vi "Set input current_ChQ.vi"(0 "channel name":string, 3 "4070_address":refnum<k15>="PXI3Slot5_5 (8)" caption="4070_out", 4 "res(input)":dbl=110.0, 6 "the optimum current(input)":dbl format="%#_6f", 7 "accuracy (input)":dbl step=0.01, 8 "instrument handle":refnum<k15>, 9 "the upper limit for the voltage":dbl=5.0, 10 "Start voltage":dbl=3.0 format="%#.7f", 11 "the lower limit for the voltage":dbl=1.0) -> (1 "current value, mA":dbl, 2 "Error message":string, 5 "accommodated voltage (out)":dbl)   [LabVIEW 2013]
uses:
  <instrlib>/niDMM/nidmm.llb/niDMM Resolution in Digits.ctl
  <instrlib>/niDMM/nidmm.llb/niDMM Function.ctl
  <vilib>/Analysis/baseanly.llb/Mean (DBL).vi
  <instrlib>/niDMM/nidmm.llb/niDMM Configure Measurement Digits.vi
  <vilib>/Analysis/NI_AALBase.lvlib
panel:
  out "CH1_Uпит, mA":dbl=15.418111291908591 caption="CH1_AO, ìA" format="%_6g"
  out "the voltage drop across the resistor":dbl=1.1
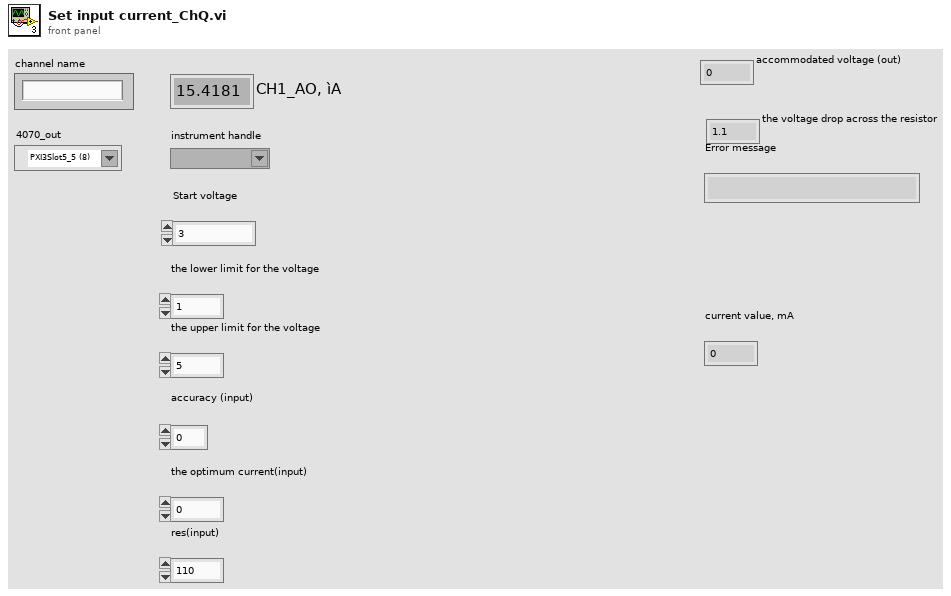
[diagram p1: front panel]
types:
  T1 = typedef "niDMM Function.ctl" = enum16{"DC Volts", "AC Volts", "DC Current", "AC Current", "2-wire Resistance", "4-wire Resistance", "Diode", "Frequency", "Period", "AC Volts DC Coupled", "Capacitance", "Inductance", "Temperature"}
  T2 = typedef "niDMM Resolution in Digits.ctl" = dbl
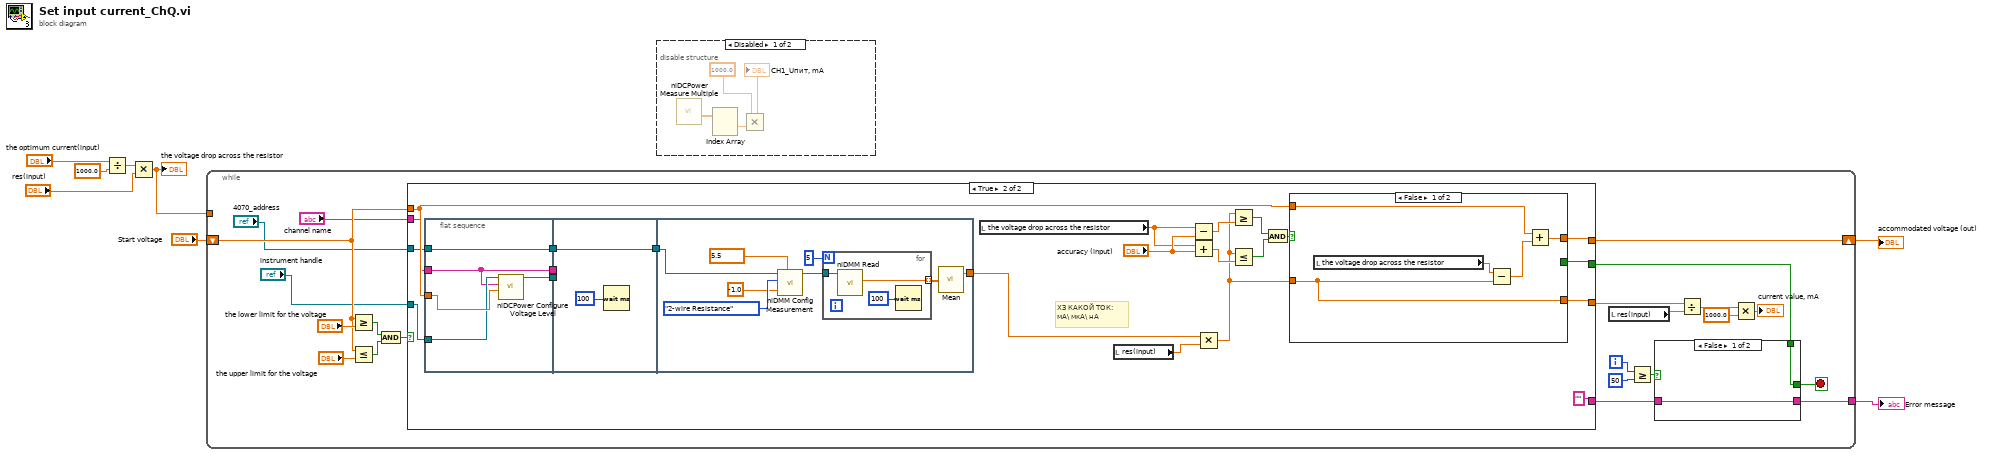
[diagram p0: block diagram]
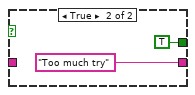
[diagram p3: hidden frame]
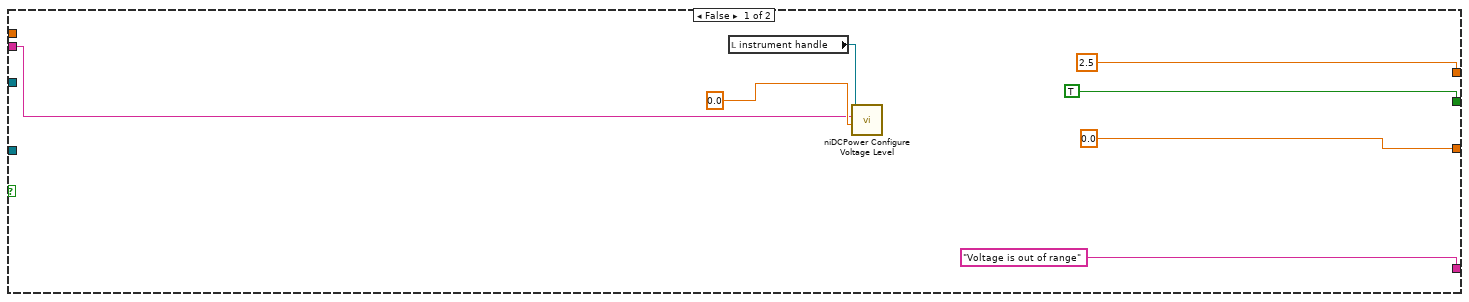
[diagram p4: hidden frame]
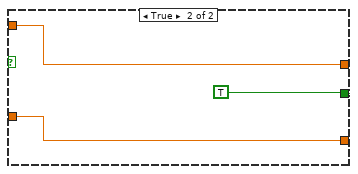
[diagram p5: hidden frame]
diagram:
  n1 = Divide(x="the optimum current(input)", y=1000.0) -> (x/y=w5:dbl)
  n2 = Multiply(x=w5, y="res(input)") -> (x*y=w1:dbl)
  "the voltage drop across the resistor" <- w1
  n3 = while {
    tunnel: [w14] -> w8
    shift-right: [w20] -> w2
    shift-left: "Start voltage" -> [w21]
    tunnel: w1 -> [_]
    i -> [w17]
    stop <- w13 stop-if-true
    n4 = Greater Or Equal?(x=w21, y="the lower limit for the voltage") -> (x >= y?=w29:bool)
    n5 = Less Or Equal?(x=w21, y="the upper limit for the voltage") -> (x <= y?=w30:bool)
    n6 = And(x=w29, y=w30) -> (x .and. y?=w26:bool)
    n7 = case shown="True" w26 {
      tunnel: ["Voltage is out of range" ""] -> w15
      tunnel: [2.5 ("accommodated voltage") w55] -> w20
      tunnel: [TRUE w61] -> w12
      tunnel: [0.0 w56] -> w19
      tunnel: w21 -> [_ w51]
      tunnel: "instrument handle" -> [_ w47]
      tunnel: "channel name" -> [w35 w46]
      tunnel: "4070_address" -> [_ w44]
      frame False {
        n8 = local read "instrument handle"() -> (w37:refnum<k15>)
        n9 = call <instrlib>:"niDCPower Configure Voltage Level.vi"("voltage level"=0.0, "channel name"=w35, "instrument handle"=w37) -> ()  [unwired: 7 in, 2 out]
      }
      frame True {
        # "ХЗ КАКОЙ ТОК:\nмА\\ мкА\\ нА"
        n10 = flat-sequence {
          tunnel: w51 -> [w67]
          tunnel: [w68] -> w52
          tunnel: [w65] -> w48
          tunnel: w47 -> [w66]
          tunnel: w46 -> [w65]
          tunnel: [w64] -> w45
          tunnel: w44 -> [w64]
          tunnel: w52 -> [_]
          tunnel: w48 -> [_]
          tunnel: w45 -> [w69]
          tunnel: [w69] -> w43
          tunnel: w43 -> [w72]
          tunnel: [w71] -> w42
          frame #0 {
            n11 = call <instrlib>:"niDCPower Configure Voltage Level.vi"("voltage level"=w67, "channel name"=w65, "instrument handle"=w66) -> ("instrument handle out"=w68:refnum<k15>)  [unwired: 7 in, 1 out]
          }
          frame #1 {
            n12 = Wait (ms)(milliseconds to wait=u32 100) -> ()  [unwired: 1 out]
          }
          frame #2 {
            w75 = T2 5.5 items=["3 1/2"=3.5, "4 1/2"=4.5, "5 1/2"=5.5, "6 1/2"=6.5, "7 1/2"=7.5] ("Resolution in Digits")
            n13 = call-poly <instrlib>:"niDMM Config Measurement.vi"("Range"=-1.0 ("Configuration:Measurement Options:Max Frequency"), "Resolution in Digits"=w75, "Function"=niDMM_Function."2-wire Resistance" ("multimeter mode"), "instrument handle"=w72) -> ("instrument handle out"=w76:refnum<k15>)  [unwired: 6 in, 1 out]
            n14 = for {
              N: 5 -> [_]
              tunnel: w76 -> [w80]
              tunnel: [w79] -> w77 mode=indexing
              n15 = call <instrlib>:"niDMM Read.vi"("instrument handle"=w80) -> ("Measurement"=w79:dbl)  [unwired: 8 in, 2 out]
              n16 = Wait (ms)(milliseconds to wait=u32 100) -> ()  [unwired: 1 out]
            }
            n17 = call-poly <vilib>:"Mean.vi"("X"=w77) -> ("mean"=w71:dbl)  [unwired: 1 out]
          }
        }
        n18 = local read "the voltage drop across the resistor"() -> (w59:dbl)
        n19 = local read "res(input)"() -> (w50:dbl)
        n20 = Subtract(x=w59, y="accuracy (input)") -> (x-y=w63:dbl)
        n21 = Add(x=w59, y="accuracy (input)") -> (x+y=w62:dbl)
        n22 = Multiply(x=w42, y=w50) -> (x*y=w49:dbl)
        n23 = Greater Or Equal?(x=w49, y=w63) -> (x >= y?=w57:bool)
        n24 = Less Or Equal?(x=w49, y=w62) -> (x <= y?=w58:bool)
        n25 = And(x=w57, y=w58) -> (x .and. y?=w54:bool)
        n26 = case shown="False" w54 {
          tunnel: [_ TRUE] -> w61
          tunnel: [w85 w87] -> w55
          tunnel: w49 -> [w83 w88]
          tunnel: [w83 w88] -> w56
          tunnel: w51 -> [w84 w87]
          frame False {
            n27 = local read "the voltage drop across the resistor"() -> (w82:dbl)
            n28 = Subtract(x=w82, y=w83) -> (x-y=w86:dbl)
            n29 = Add(x=w84, y=w86) -> (x+y=w85:dbl)
          }
          frame True {
          }
        }
      }
    }
    n30 = local read "res(input)"() -> (w25:dbl)
    n31 = Greater Or Equal?(x=w17, y=50) -> (x >= y?=w18:bool)
    n32 = case shown="False" w18 {
      tunnel: w15 -> [w32 _]
      tunnel: [w32 "Too much try"] -> w14
      tunnel: [w31 TRUE] -> w13
      tunnel: w12 -> [w31 _]
      frame False {
      }
      frame True {
      }
    }
    n33 = Divide(x=w19, y=w25) -> (x/y=w24:dbl)
    n34 = Multiply(x=w24, y=1000.0) -> (x*y=→"current value, mA":dbl)
  }
  "Error message" <- w8
  "accommodated voltage (out)" <- w2
  n35 = disable-structure shown="Disabled" {
    frame Disabled {
      n36 = call <instrlib>:"niDCPower Measure Multiple.vi"() -> ("current measurements"=w90:dbl[])  [unwired: 8 in, 3 out]
      n37 = Index Array(array=w90) -> (element #1=w92:dbl)  [unwired: 2 in, 1 out]
      n38 = Multiply(x=1000.0 ("y"), y=w92) -> (x*y=→"CH1_Uпит, mA":dbl)
    }
    frame Enabled {
    }
  }
